vi "Load.vi"(8 "error in (no error)":errorcluster, 11 "Test Configs In":T1) -> (0 "error out":errorcluster, 3 "Test Configs Out":T1)   [LabVIEW 2015]
doc: "Load a test configuration into the front panel control"
uses:
  Type Defs/Sequence Parameters Ref.ctl
  Type Defs/Sequence Parameters.ctl
  Type Defs/Target Type.ctl
  Type Defs/Variable Data Type.ctl
  <vilib>/Utility/xml.llb/Read From XML File(string).vi
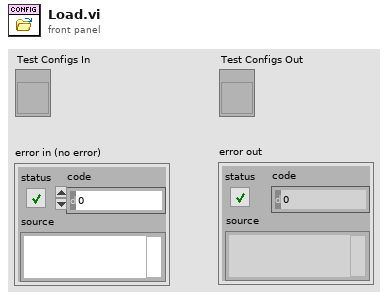
[diagram p1: front panel]
types:
  T1 = typedef "Sequence Parameters Ref.ctl" = refnum<vi>
  T2 = enum16{"open", "replace", "create", "open or create", "replace or create", "replace or create with confirmation"}
  T3 = typedef "Sequence Parameters.ctl" = cluster{"Test Name":string, "Target":T4, "Host IP Address":string, "Target IP Address":string, "Shared Variable Host":enum16{"Target", "Host"}, "Shared Variable Writer":enum16{"Target", "Host"}, "Variable Data Type":T5, "# of Variables per Library":u16, "Update Rate (Hz)":dbl, "Read Rate (Hz)":dbl, "Floor":u32, "Ceiling":u32, "Delta":u32}
  T4 = typedef "Target Type.ctl" = enum16{"cRIO-9012", "cRIO-9014", "cRIO-9022", "cRIO-9023", "cRIO-9024", "cRIO-9025", "cRIO-9068", "cRIO-9073", "cRIO-9074", "cRIO-9075", "cRIO-9076", "cRIO-9081", "cRIO-9082", "myRIO-1900", "myRIO-1950", "PXI-8101", "PXI-8115", "PXI-8119", "PXI-8820", "PXIe-8100", "PXIe-8101", "PXIe-8133", "PXIe-8135", "PXIe-8820", "sbRIO-9605", "sbRIO-9606", "sbRIO-9623", "sbRIO-9626", "sbRIO-9633", "sbRIO-9636", "Unlisted (Linux-RT)", "Unlisted (PharLap)", "Unlisted (VxWorks)", "Windows Target"}
  T5 = typedef "Variable Data Type.ctl" = enum16{"U8", "U16", "U32", "U64", "I8", "I16", "I32", "I64", "Single", "Double", "Boolean", "String"}
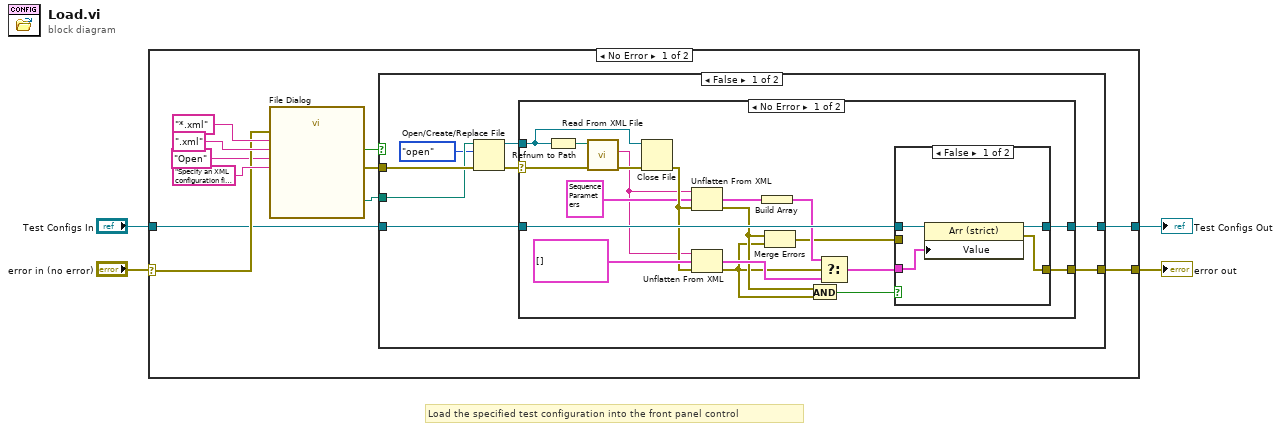
[diagram p0: block diagram]
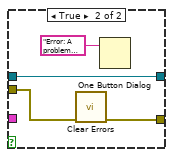
[diagram p2: hidden frame]
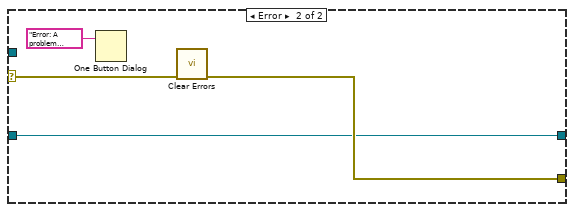
[diagram p3: hidden frame]
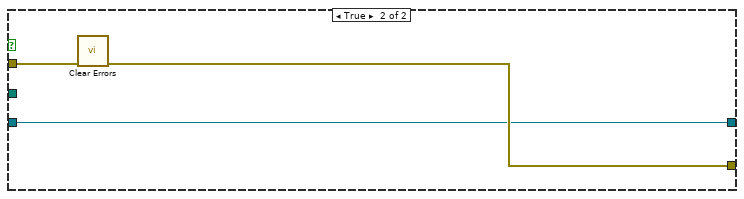
[diagram p4: hidden frame]
diagram:
  # "Load the specified test configuration into the front panel control"
  n1 = case shown="No Error" "error in (no error)" {
    selector: "error in (no error)" -> [w9 w58]
    tunnel: "Test Configs In" -> [w7 w59]
    tunnel: [w6 w59] -> w1
    tunnel: [w5 w58] -> w3
    frame No Error {
      n2 = call "File Dialog"("prompt"="Specify an XML configuration file to open", "button label"="Open", "error in"=w9, "pattern (all files)"="*.xml", "pattern label"=".xml" ("pattern (all files)")) -> ("selected path"=w12:path, "cancelled"=w14:bool, "error out"=w13:errorcluster)  [unwired: 7 in, 1 out]
      n3 = case shown="False" w14 {
        tunnel: w13 -> [w23 w57]
        tunnel: w12 -> [w22 _]
        tunnel: w7 -> [w18 w55]
        tunnel: [w17 w55] -> w6
        tunnel: [w16 w56] -> w5
        frame False {
          n4 = Open/Create/Replace File(file path (use dialog)=w22, error in=w23, operation (0:open)=T2."open") -> (refnum out=w19:refnum<file>, error out=w20:errorcluster)  [unwired: 3 in, 1 out]
          n5 = case shown="No Error" w20 {
            selector: w20 -> [w41 w54]
            tunnel: w19 -> [w40 _]
            tunnel: w18 -> [w36 w51]
            tunnel: [w35 w51] -> w17
            tunnel: [w37 w52] -> w16
            frame No Error {
              n6 = Refnum to Path(1:w40) -> (0:w42:path)
              n7 = call-poly <vilib>:"Read From XML File.vi"("error in (no error)"=w41, "XML File Path"=w42) -> ("error out"=w39:errorcluster, "XML Elements"=w24:string)  [unwired: 7 in, 1 out]
              n8 = Close File(refnum=w40, error in=w39) -> (error out=w34:errorcluster)  [unwired: 1 out]
              n9 = Unflatten From XML(xml string=w24, type=T3 {"Test Name"="Unique Test Name", "Target"=enum."cRIO-9012", "Host IP Address"="0.0.0.0", "Target IP Address"="0.0.0.0", "Shared Variable Host"=enum."Target", "Shared Variable Writer"=enum."Target", "Variable Data Type"=enum."Double", "# of Variables per Library"=500, "Update Rate (Hz)"=1.0, "Read Rate (Hz)"=1.0, "Floor"=500, "Ceiling"=5000, "Delta"=500} ("Test Parameters"), error in (no error)=w34) -> (value=w32:T3, error out=w29:errorcluster)
              n10 = Unflatten From XML(xml string=w24, type=T3[] [], error in (no error)=w34) -> (value=w31:T3[], error out=w28:errorcluster)
              n11 = Build Array(w32) -> (w30:T3[])
              n12 = Merge Errors(w29, w28) -> (w25:errorcluster)
              n13 = And(x=w29, y=w28) -> (x .and. y?=w26:bool)
              n14 = Select(t=w30, s=w28, f=w31) -> (s? t:f=w27:T3[])
              n15 = case shown="False" w26 {
                tunnel: w27 -> [w45 _]
                tunnel: [w44 w50] -> w37
                tunnel: w36 -> [w46 w48]
                tunnel: [w43 w48] -> w35
                tunnel: w25 -> [_ w47]
                frame False {
                  n16 = property class="Arr (strict)"(reference=w46, "Value"=w45) -> (reference out=w43:T1, error out=w44:errorcluster)  [unwired: 1 in]
                }
                frame True {
                  n17 = call <vilib>:"Clear Errors.vi"("error in (no error)"=w47) -> ("error out"=w50:errorcluster)  [unwired: 5 in, 1 out]
                  n18 = One Button Dialog(message="Error: A problem occured while parsing the test configuration file. Ensure the file selected is a valid XML test configuration file created by this tool. ") -> ()  [unwired: 1 in, 1 out]
                }
              }
            }
            frame Error {
              n19 = One Button Dialog(message="Error: A problem occured while opening the test configuration file. Ensure the path selected leads to a valid XML test configuration file.") -> ()  [unwired: 1 in, 1 out]
              n20 = call <vilib>:"Clear Errors.vi"("error in (no error)"=w54) -> ("error out"=w52:errorcluster)  [unwired: 5 in, 1 out]
            }
          }
        }
        frame True {
          n21 = call <vilib>:"Clear Errors.vi"("error in (no error)"=w57) -> ("error out"=w56:errorcluster)  [unwired: 5 in, 1 out]
        }
      }
    }
    frame Error {
    }
  }
  "error out" <- w3
  "Test Configs Out" <- w1
